vi "Download File.vi"(6 "timeout (ms)":i32=30000, 8 "error in":errorcluster, 9 "local path":path, 10 "remote path":string, 11 "session in":refnum<class "Session.lvclass">) -> (0 "error out":errorcluster, 3 "session out":refnum<class "Session.lvclass">)   [LabVIEW 2020, in "NI_SFTP.lvlib"]
doc: "Downloads a remote file, storing the contents in a local file."
uses:
  <vilib>/net/SFTP/NI_SFTP.lvlib
  <vilib>/net/SFTP/Session/Session.lvclass
  <vilib>/net/SFTP/Session/Session.lvclass/Session.ctl
  <vilib>/net/SFTP/Session/Read fsync.vi
  <vilib>/net/SFTP/API/Support/Download/File/File Download Controller.lvclass
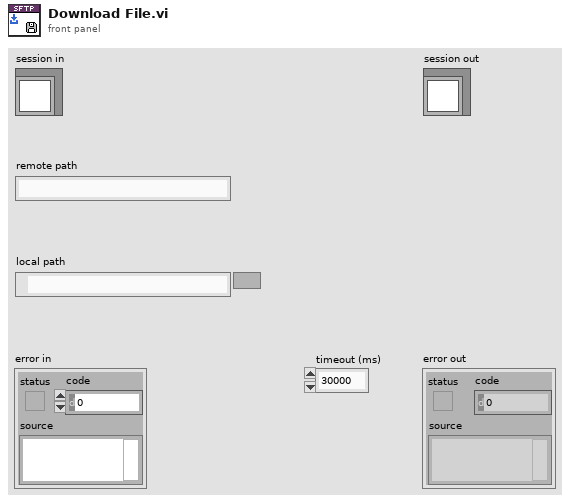
[diagram p1: front panel]
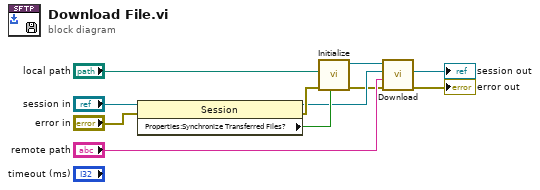
[diagram p0: block diagram]
diagram:
  n1 = property on="Property Node" class="Session"(reference="session in", error in="error in") -> (reference out=w5:refnum<class "Session.lvclass">, error out=w8:errorcluster, "Properties:Synchronize Transferred Files?"=w7:bool)
  n2 = call <vilib>:"Initialize.vi"("Synchronize Transferred Files"=w7, "error in (no error)"=w8, "local path"="local path") -> ("error out"=w3:errorcluster, "File Download Controller out"=w6:refnum<class "File Download Controller.lvclass">)  [unwired: 7 in]
  n3 = call-dynamic "Download.vi"("error in"=w3, "remote path"="remote path", "session in"=w5, "NI_SFTP.lvlib:Generic Download Controller.lvclass"=w6) -> ("error out"=→"error out":errorcluster, "session out"=→"session out":refnum<class "Session.lvclass">)  [unwired: 5 in, 1 out]
